vi "svl_Impulse Peak Detector with IC.vi"(2 "init/cont (init:F)":bool, 3 "initial filter state":dbl format="%.2f", 4 "sampling frequency [Hz]":dbl=10000.0 format="%.2f", 5 "X":dbl[](array[numeric]) format="%.2f") -> (0 "final filter state":dbl format="%.2f", 1 "filtered X":dbl[](array[numeric]) format="%.2f")   [LabVIEW 2017]
doc: "Detects peaks with a decay time constant of 1500 ms on the input signal X and returns the entire filtered signal.\nThe initial filter state and the final filter state parameters keep track of the internal state of the filter to ensure continuous operation of the filter if continuous mode is used."
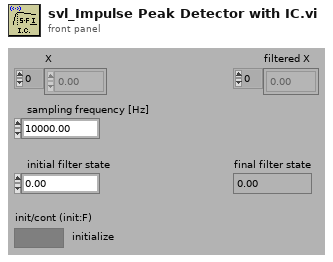
[diagram p1: front panel]
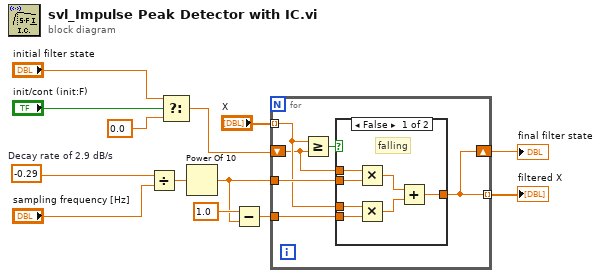
[diagram p0: block diagram]
diagram:
  w13 = -0.29  # Decay rate of 2.9 dB/s
  n1 = Divide(x=w13, y="sampling frequency [Hz]") -> (x/y=w11:dbl)
  n2 = Select(t="initial filter state", s="init/cont (init:F)", f=0.0) -> (s? t:f=w1:dbl)
  n3 = Power Of 10(x=w11) -> (10^x=w8:dbl)
  n4 = Subtract(x=1.0, y=w8) -> (x-y=w7:dbl)
  n5 = for {
    tunnel: "X" -> [w16] mode=indexing
    tunnel: w8 -> [w19]
    tunnel: w7 -> [w18]
    shift-right: [w15] -> w5
    shift-left: w1 -> [w14]
    tunnel: [w15] -> w6 mode=indexing
    n6 = Greater Or Equal?(x=w16, y=w14) -> (x >= y?=w17:bool)
    n7 = case shown="False" w17 {
      tunnel: w19 -> [w24 _]
      tunnel: w18 -> [w23 _]
      tunnel: w16 -> [w22 w27]
      tunnel: w14 -> [w21 _]
      tunnel: [w20 w27] -> w15
      frame False {
        # "falling"
        n8 = Multiply(x=w21, y=w24) -> (x*y=w25:dbl)
        n9 = Multiply(x=w22, y=w23) -> (x*y=w26:dbl)
        n10 = Add(x=w25, y=w26) -> (x+y=w20:dbl)
      }
      frame True {
        # "rising"
      }
    }
  }
  "filtered X" <- w6
  "final filter state" <- w5
